vi "CTRE_Tank_RefNumRegistryGet.vi"(10 "RefNum Name":string) -> (3 "Tank Drivetrain":T1)   [LabVIEW 2016]
uses:
  <vilib>/Rock Robotics/WPI/ThirdParty/CanMotor/CTRLib-LV-TalonSRX/Framework/Tank.ctl
  <vilib>/Rock Robotics/WPI/MotorControl/WPI_MotorControlDeviceRef.ctl
  <vilib>/Rock Robotics/WPI/MotorControl/WPI_MotorControlType.ctl
  <vilib>/Rock Robotics/SystemInterfaces/DIO/FPGA_DIOPWMChannel.ctl
  <vilib>/Rock Robotics/WPI/PWM/WPI_PWMDeadband.ctl
  <vilib>/Rock Robotics/WPI/Utilities/Refnum Registry Operation.ctl
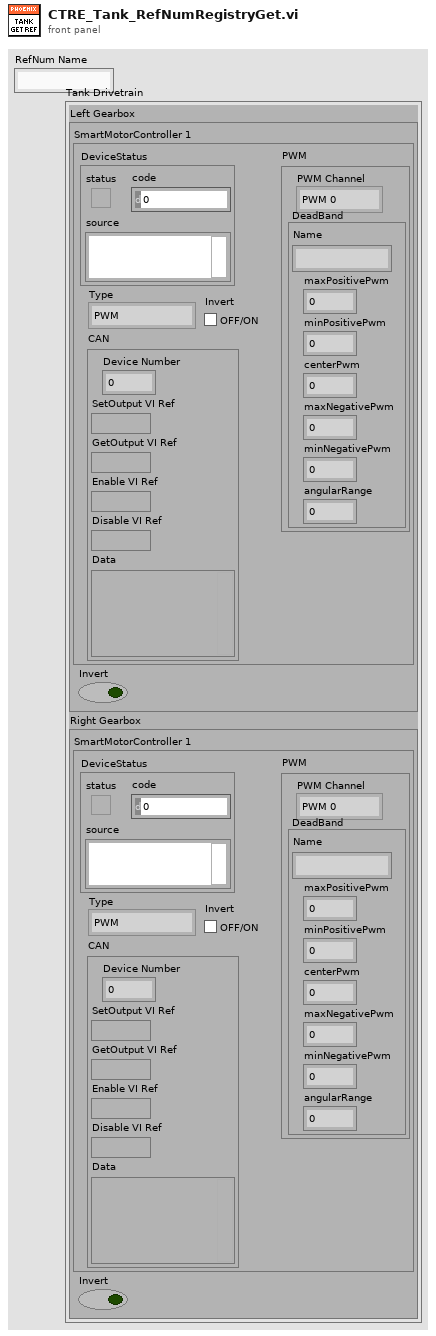
[diagram p1: front panel]
types:
  T1 = typedef "Tank.ctl" = cluster{"Left Gearbox":cluster{"SmartMotorController 1":T2, "Invert":bool}, "Right Gearbox":cluster{"SmartMotorController 1":T2, "Invert":bool}}
  T2 = typedef "WPI_MotorControlDeviceRef.ctl" = cluster{"DeviceStatus":errorcluster, "Type":T3, "PWM":cluster{"PWM Channel":T4, "DeadBand":T5}, "CAN":cluster{"Device Number":u8, "SetOutput VI Ref":variant, "GetOutput VI Ref":variant, "Enable VI Ref":variant, "Disable VI Ref":variant, "Data":variant}, "Invert":bool}
  T3 = typedef "WPI_MotorControlType.ctl" = enum16{"PWM", "CAN"}
  T4 = typedef "FPGA_DIOPWMChannel.ctl" = enum8{"PWM 0", "PWM 1", "PWM 2", "PWM 3", "PWM 4", "PWM 5", "PWM 6", "PWM 7", "PWM 8", "PWM 9", "PWM MXP 0", "PWM MXP 1", "PWM MXP 2", "PWM MXP 3", "PWM MXP 4", "PWM MXP 5", "PWM MXP 6", "PWM MXP 7", "PWM MXP 8", "PWM MXP 9", "Invalid"}
  T5 = typedef "WPI_PWMDeadband.ctl" = cluster{"Name":string, "maxPositivePwm":i32, "minPositivePwm":i32, "centerPwm":i32, "maxNegativePwm":i32, "minNegativePwm":i32, "angularRange":u16}
  T6 = typedef "Refnum Registry Operation.ctl" = enum16{"set", "get", "delete", "get all names", "read name"}
  T7 = cluster{"Left Gearbox":cluster{"SmartMotorController 1":T2, "Invert":bool}, "Right Gearbox":cluster{"SmartMotorController 1":T2, "Invert":bool}}
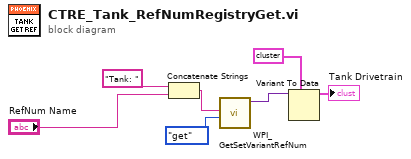
[diagram p0: block diagram]
diagram:
  n1 = Concatenate Strings("Tank: " ("string"), "RefNum Name") -> (w5:string)
  n2 = call <vilib>:"WPI_GetSetVariantRefNum.vi"("Operation"=Refnum_Registry_Operation."get", "refnum name"=w5) -> ("DevRef"=w2:variant)  [unwired: 7 in, 2 out]
  n3 = Variant To Data(type=T7 {"Left Gearbox"={"SmartMotorController 1"={"DeviceStatus"={"status"=FALSE, "code"=0, "source"=""}, "Type"=enum."PWM", "PWM"={"PWM Channel"=enum."PWM 1", "DeadBand"={"Name"="", "maxPositivePwm"=0, "minPositivePwm"=0, "centerPwm"=0, "maxNegativePwm"=0, "minNegativePwm"=0, "angularRange"=0}}, "CAN"={"Device Number"=0, "SetOutput VI Ref"=variant(enum8{"Percent VBus", "Current", "Speed", "Position", "Voltage"} enum."Percent VBus"), "GetOutput VI Ref"=variant(refnum<k1> refnum), "Enable VI Ref"=variant(dbl 12.0), "Disable VI Ref"=variant(enum8{"Percent VBus", "Speed", "Position", "Slave", "Unchanged / Invalid", "Voltage Compensation", "Current", "Motion Profile"} enum."Percent VBus"), "Data"=variant}, "Invert"=FALSE}, "Invert"=FALSE}, "Right Gearbox"={"SmartMotorController 1"={"DeviceStatus"={"status"=FALSE, "code"=0, "source"=""}, "Type"=enum."PWM", "PWM"={"PWM Channel"=enum."PWM 1", "DeadBand"={"Name"="", "maxPositivePwm"=0, "minPositivePwm"=0, "centerPwm"=0, "maxNegativePwm"=0, "minNegativePwm"=0, "angularRange"=0}}, "CAN"={"Device Number"=0, "SetOutput VI Ref"=variant(enum8{"Percent VBus", "Current", "Speed", "Position", "Voltage"} enum."Percent VBus"), "GetOutput VI Ref"=variant(refnum<k1> refnum), "Enable VI Ref"=variant(dbl 12.0), "Disable VI Ref"=variant(enum8{"Percent VBus", "Speed", "Position", "Slave", "Unchanged / Invalid", "Voltage Compensation", "Current", "Motion Profile"} enum."Percent VBus"), "Data"=variant}, "Invert"=FALSE}, "Invert"=FALSE}} ("Tank Drivetrain"), Variant=w2) -> (data=→"Tank Drivetrain":T7)  [unwired: 1 in, 1 out]
